vi "Write&ReadWord.vi"(8 "error in":errorcluster) -> (0 "error out":errorcluster, 2 "¿Esta abierto?":bool)   [LabVIEW 2019]
doc: "Este VI puede leer y escribir en un documento de Microsoft Word. Se puede switchear entre esta dos opciones en el front panel durante la ejecución"
panel:
  in  "?":bool
  in  "Escribe aquí":string="Cola"
  in  "?":bool
  out "?":string
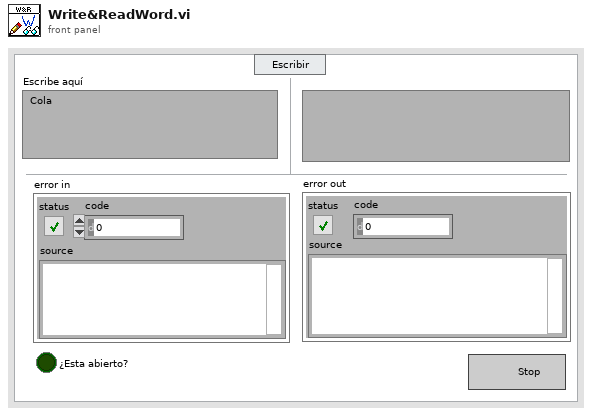
[diagram p1: front panel]
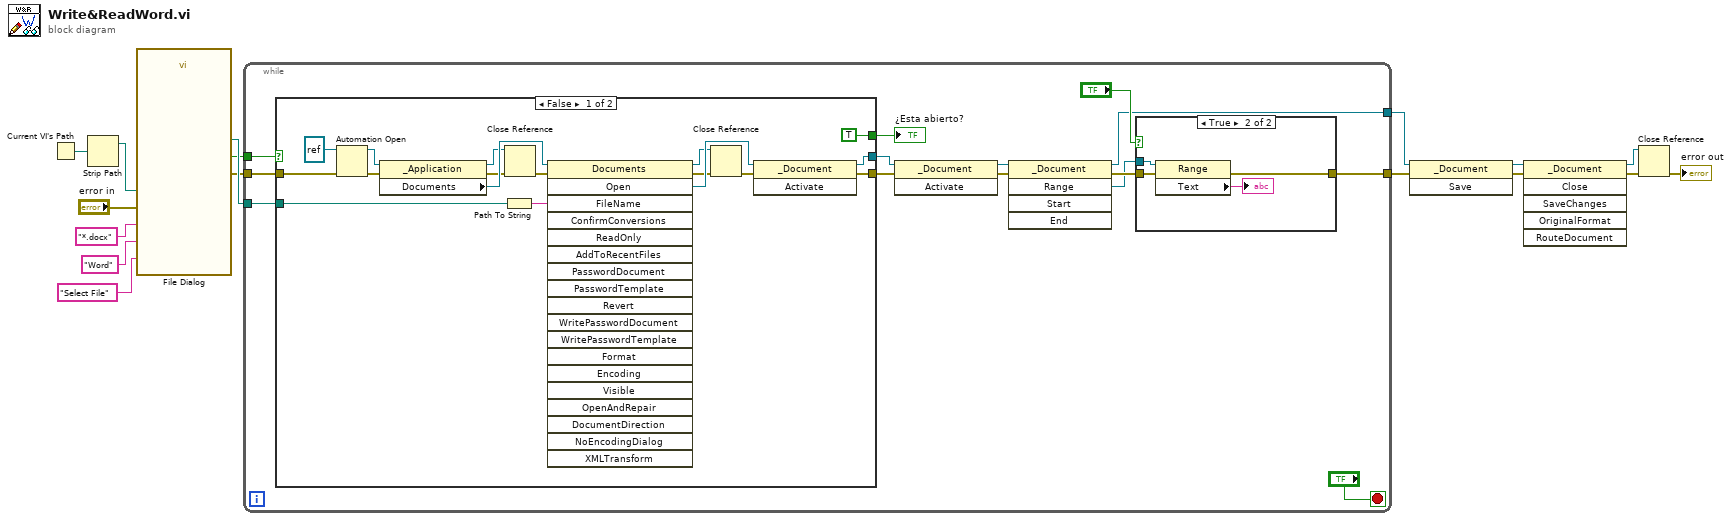
[diagram p0: block diagram]
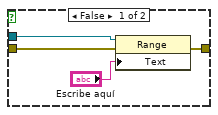
[diagram p2: hidden frame]
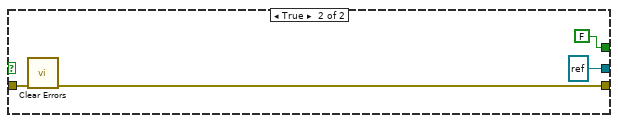
[diagram p3: hidden frame]
diagram:
  n1 = Current VI's Path() -> (path=w14:path)
  n2 = Strip Path(path=w14) -> (stripped path=w16:path)  [unwired: 1 out]
  n3 = call "File Dialog"("start path"=w16, "prompt"="Select File", "error in"="error in", "pattern (all files)"="*.docx", "pattern label"="Word") -> ("selected path"=w10:path, "cancelled"=w9:bool, "error out"=w8:errorcluster)  [unwired: 7 in, 1 out]
  n4 = while {
    tunnel: w10 -> [w21]
    tunnel: w9 -> [w20]
    tunnel: w8 -> [w19]
    tunnel: [w18] -> w7
    tunnel: [w17] -> w6
    stop <- "?" stop-if-true
    n5 = case shown="False" w20 {
      tunnel: w21 -> [w49 _]
      tunnel: w19 -> [w47 w59]
      tunnel: [TRUE FALSE] -> w30
      tunnel: [w46 w58] -> w26
      tunnel: [w43 refnum<k7> refnum ("reference out")] -> w29
      frame False {
        n6 = Automation Open(error in (no error)=w47, Automation Refnum=refnum<k7> refnum ("Word._Application")) -> (Automation Refnum=w51:refnum<k7>, error out=w52:errorcluster)  [unwired: 2 in]
        n7 = property class="_Application"(reference=w51, error in=w52) -> (reference out=w44:refnum<k7>, error out=w42:errorcluster, "Documents"=w53:refnum<k7>)
        n8 = Path To String(path=w49) -> (string=w55:string)
        n9 = Close Reference(reference=w44, error in (no error)=w42) -> (error out=w41:errorcluster)
        n10 = invoke class="Documents" method="Open"(reference=w53, error in=w41, "FileName"=w55) -> (reference out=w45:refnum<k7>, error out=w40:errorcluster, "Open"=w54:refnum<k7>)  [unwired: 16 in, 16 out]
        n11 = Close Reference(reference=w45, error in (no error)=w40) -> (error out=w39:errorcluster)
        n12 = invoke class="_Document" method="Activate"(reference=w54, error in=w39) -> (reference out=w43:refnum<k7>, error out=w46:errorcluster)  [unwired: 1 in, 1 out]
      }
      frame True {
        n13 = call <vilib>:"Clear Errors.vi"("error in (no error)"=w59) -> ("error out"=w58:errorcluster)  [unwired: 5 in, 1 out]
      }
    }
    "¿Esta abierto?" <- w30
    n14 = invoke class="_Document" method="Activate"(reference=w29, error in=w26) -> (reference out=w28:refnum<k7>, error out=w25:errorcluster)  [unwired: 1 in, 1 out]
    n15 = invoke class="_Document" method="Range"(reference=w28, error in=w25) -> (reference out=w18:refnum<k7>, error out=w27:errorcluster, "Range"=w24:refnum<k7>)  [unwired: 3 in, 2 out]
    n16 = case shown="True" "?" {
      tunnel: w27 -> [w34 w37]
      tunnel: [w33 w36] -> w17
      tunnel: w24 -> [w32 w35]
      frame False {
        n17 = property class="Range"(reference=w32, error in=w34, "Text"="Escribe aquí") -> (error out=w33:errorcluster)  [unwired: 1 out]
      }
      frame True {
        n18 = property class="Range"(reference=w35, error in=w37) -> (error out=w36:errorcluster, "Text"=→"?":string)  [unwired: 1 out]
      }
    }
  }
  n19 = invoke class="_Document" method="Save"(reference=w7, error in=w6) -> (reference out=w5:refnum<k7>, error out=w4:errorcluster)  [unwired: 1 in, 1 out]
  n20 = invoke class="_Document" method="Close"(reference=w5, error in=w4) -> (reference out=w1:refnum<k7>, error out=w3:errorcluster)  [unwired: 4 in, 4 out]
  n21 = Close Reference(reference=w1, error in (no error)=w3) -> (error out=→"error out":errorcluster)
